vi "Notifier Performance Test.vi"() -> ()   [LabVIEW 2021]
panel:
  out "Numeric 6":i32
  in  "stop 3":bool
  out "Boolean 6":bool
  in  "Boolean 5":bool
  out "Numeric 5":i32
  in  "stop 2":bool
  out "Boolean 4":bool
  in  "Boolean 3":bool
  out "timed out? 2":bool
  out "Numeric 3":i32
  out "notification 2":bool[](array[boolean])
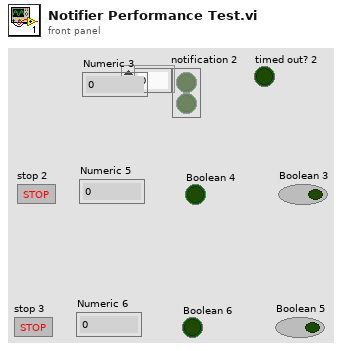
[diagram p1: front panel]
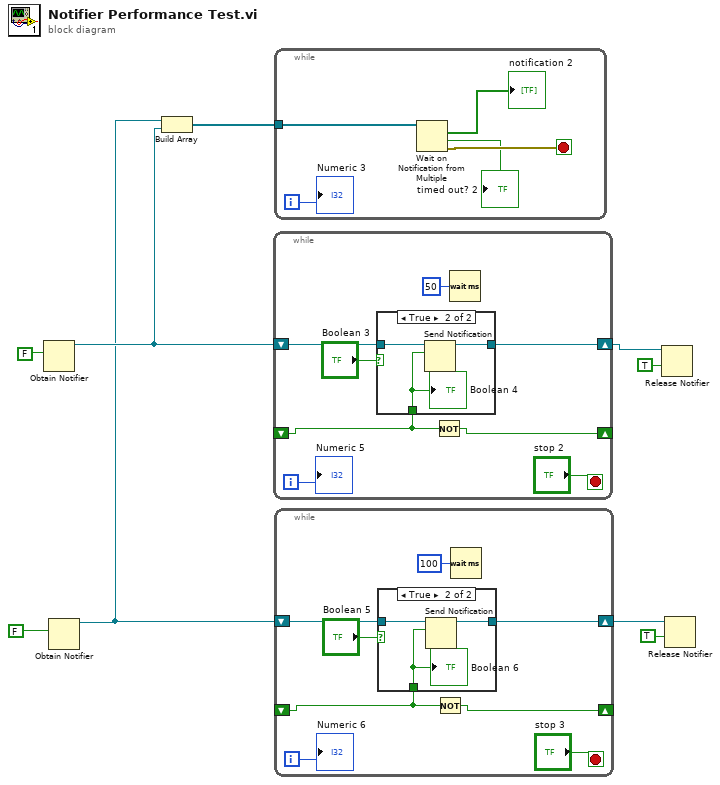
[diagram p0: block diagram]
diagram:
  n1 = Obtain Notifier(notification data type=FALSE) -> (notifier out=w7:refnum<notifier>)  [unwired: 3 in, 2 out]
  n2 = Obtain Notifier(notification data type=FALSE) -> (notifier out=w6:refnum<notifier>)  [unwired: 3 in, 2 out]
  n3 = Build Array(w6, w7) -> (w1:refnum<notifier>[])
  n4 = while {
    shift-right: [w16] -> _
    shift-left: _ -> [w15]
    shift-right: [w12] -> w4
    shift-left: w7 -> [w17]
    i -> [w14]
    stop <- "stop 2" stop-if-true
    n5 = case shown="True" "Boolean 3" {
      tunnel: w17 -> [w18 w21]
      tunnel: w15 -> [_ w19]
      tunnel: [w18 w20] -> w12
      frame False {
      }
      frame True {
        n6 = Send Notification(notification=w19, notifier=w21) -> (notifier out=w20:refnum<notifier>)  [unwired: 1 in, 1 out]
        "Boolean 4" <- w19
      }
    }
    n7 = Not(x=w15) -> (.not. x?=w16:bool)
    n8 = Wait (ms)(milliseconds to wait=u32 50) -> ()  [unwired: 1 out]
    "Numeric 5" <- w14
  }
  n9 = while {
    tunnel: w1 -> [w22]
    i -> [w26]
    stop <- w24 stop-if-true
    n10 = Wait on Notification from Multiple(0:w22) -> (9:→"notification 2":bool[], 10:→"timed out? 2":bool, 11:w24:errorcluster)  [unwired: 3 in, 1 out]
    "Numeric 3" <- w26
  }
  n11 = while {
    shift-right: [w33] -> _
    shift-left: _ -> [w32]
    shift-right: [w29] -> w2
    shift-left: w6 -> [w34]
    i -> [w31]
    stop <- "stop 3" stop-if-true
    n12 = case shown="True" "Boolean 5" {
      tunnel: w34 -> [w35 w38]
      tunnel: w32 -> [_ w36]
      tunnel: [w35 w37] -> w29
      frame False {
      }
      frame True {
        n13 = Send Notification(notification=w36, notifier=w38) -> (notifier out=w37:refnum<notifier>)  [unwired: 1 in, 1 out]
        "Boolean 6" <- w36
      }
    }
    n14 = Not(x=w32) -> (.not. x?=w33:bool)
    n15 = Wait (ms)(milliseconds to wait=u32 100) -> ()  [unwired: 1 out]
    "Numeric 6" <- w31
  }
  n16 = Release Notifier(notifier=w4, force destroy? (F)=TRUE) -> ()  [unwired: 1 in, 3 out]
  n17 = Release Notifier(notifier=w2, force destroy? (F)=TRUE) -> ()  [unwired: 1 in, 3 out]
